vi "Delete Certificate.vi"(8 "error in (no error)":errorcluster, 10 "Certificate ID":string, 11 "IoT Session in":refnum<class "IoT Session.lvclass">) -> (0 "error out":errorcluster, 3 "IoT Session out":refnum<class "IoT Session.lvclass">)   [LabVIEW 2015, in "NI_AWS_IoT.lvlib" / "IoT Session.lvclass"]
uses:
  IoT Session.lvclass
  Core/HTTP Request/Request Options.ctl
  Core/HTTP Request/Name Value Pair.ctl
  Core/HTTP Request/Region handling.ctl
  Core/HTTP Request/URL formatting.ctl
  Core/HTTP Request/HTTP Request.lvclass
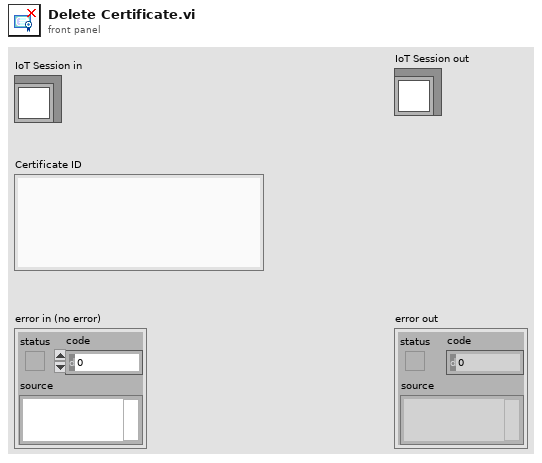
[diagram p1: front panel]
types:
  T1 = typedef "NI_AWS_Core.lvlib/HTTP Request.lvclass/Name Value Pair.ctl" = cluster{"name":string, "value":string}
  T2 = typedef "NI_AWS_Core.lvlib/HTTP Request.lvclass/Request Options.ctl" = cluster{"request headers":T1[], "request parameters":T1[], "request body":string, "region handling":T3, "URL formatting":T4}
  T3 = typedef "NI_AWS_Core.lvlib/HTTP Request.lvclass/Region handling.ctl" = enum16{"use region everywhere", "use region (authentication only)", "use region (URL only)", "ignore region everwhere"}
  T4 = typedef "NI_AWS_Core.lvlib/HTTP Request.lvclass/URL formatting.ctl" = enum16{"region-", "region."}
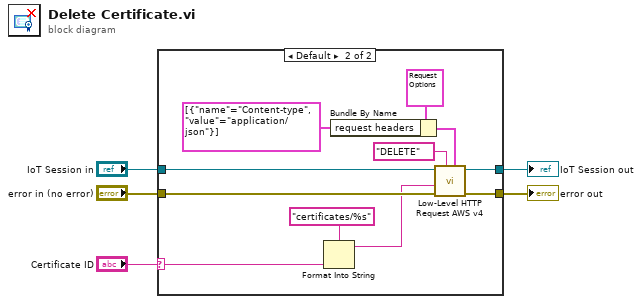
[diagram p0: block diagram]
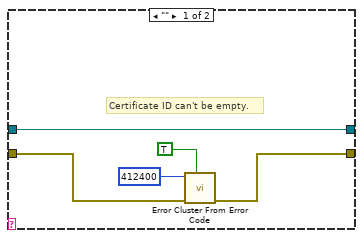
[diagram p2: hidden frame]
diagram:
  n1 = case shown="Default" "Certificate ID" {
    selector: "Certificate ID" -> [_ w12]
    tunnel: "error in (no error)" -> [w7 w21]
    tunnel: [w6 w20] -> w4
    tunnel: [w10 w19] -> w3
    tunnel: "IoT Session in" -> [w10 w18]
    frame "" {
      # "Certificate ID can't be empty."
      n2 = call <vilib>:"Error Cluster From Error Code.vi"("show call chain? (False)"=TRUE, "error in (no error)"=w7, "error code (0)"=412400) -> ("error out"=w6:errorcluster)  [unwired: 6 in]
    }
    frame Default {
      n3 = Format Into String(format string="certificates/%s", w12) -> (resulting string=w11:string)  [unwired: 2 in, 1 out]
      n4 = Bundle By Name(cluster=T2 {"request headers"=[], "request parameters"=[], "request body"="", "region handling"=enum."use region everywhere", "URL formatting"=enum."region."} ("Request Options"), "request headers"=T1[] [{"name"="Content-type", "value"="application/json"}]) -> (w15:T2)
      n5 = call "Low-Level HTTP Request AWS v4.vi"("Request Options"=w15, "HTTP-Verb"="DELETE", "error in (no error)"=w21, "URL Suffix"=w11, "AWS Core in"=w18) -> ("error out"=w20:errorcluster, "AWS Core out"=w19:refnum<class "IoT Session.lvclass">)  [unwired: 3 in, 2 out]
    }
  }
  "error out" <- w4
  "IoT Session out" <- w3
